vi "Create Map from Identifiers to Indexes.vi"(11 "RT hardware channel data":T2[](array[typedef]) {"labels settings for RT"."Label Timestamp Channel Data Reference" format="%.0x"; "labels settings for RT"."Word Initial Raw Value" format="%032.0f"; "labels settings for RT"."Label Disable/Trigger Channel Reference" format="%.0x"; "labels settings for RT"."parameter driver data"."Tx parameter refs" format="%.0x"; "labels settings for RT"."SDI" format="%02b"; "labels settings for RT"."label" format="%.0o"}) -> (3 "map from identifiers to indexes":T1)   [LabVIEW 2020, in "AIM ARINC 429 Engine.lvlib" / "Custom Device.lvlib"]
uses:
  Custom Device.lvlib
  Shared/RT Hardware Channel Settings.ctl
  Shared/RT Label Settings.ctl
  Shared/Label.ctl
  Shared/RT Parameters.ctl
  Shared/Parameter Definition.ctl
  <vilib>/NI/NI VeriStand Encoding and Decoding/Encoding.ctl
  <vilib>/NI VeriStand/Custom Device API/Custom Device Item Ref.ctl
  Shared/Transfer Type.ctl
  <vilib>/NI VeriStand/Custom Device API/Data Reference.ctl
  Shared/Map of Identifiers to Indexes.ctl
  <vilib>/NI/NI VeriStand Encoding and Decoding/Encoding and Decoding.lvlib
  <vilib>/NI VeriStand/Custom Device API/Custom Device API.lvlib
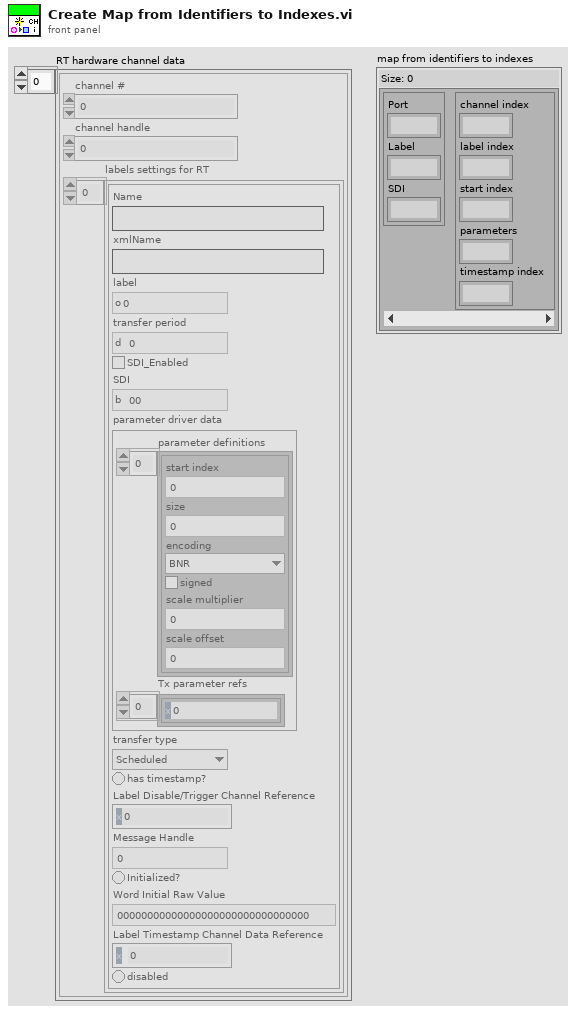
[diagram p1: front panel]
types:
  T1 = typedef "Map of Identifiers to Indexes.ctl" = map{cluster{"Port":u8, "Label":u8, "SDI":u8}, cluster{"channel index":i32, "label index":i32, "start index":i32, "parameters":i32, "timestamp index":i32}}
  T2 = typedef "RT Hardware Channel Settings.ctl" = cluster{"channel #":u16, "channel handle":u64, "labels settings for RT":T3[]}
  T3 = typedef "RT Label Settings.ctl" = cluster{"Name":string, "xmlName":string, "label":T4, "transfer period":u32, "SDI_Enabled":bool, "SDI":u8, "parameter driver data":T5, "transfer type":T9, "has timestamp?":bool, "Label Disable/Trigger Channel Reference":T8, "Message Handle":u64, "Initialized?":bool, "Word Initial Raw Value":u32, "Label Timestamp Channel Data Reference":T10, "disabled":bool}
  T4 = typedef "Label.ctl" = u8
  T5 = typedef "RT Parameters.ctl" = cluster{"parameter definitions":T6[], "Tx parameter refs":T8[]}
  T6 = typedef "Parameter Definition.ctl" = cluster{"start index":i32, "size":i32, "encoding":T7, "signed":bool, "scale multiplier":dbl, "scale offset":dbl}
  T7 = typedef "Encoding and Decoding.lvlib/Encoding.ctl" = enum16{"BNR", "BCD", "Discrete"}
  T8 = typedef "Custom Device API.lvlib/Custom Device Item Ref.ctl" = u64
  T9 = typedef "Transfer Type.ctl" = enum16{"Scheduled", "Acyclic", "Block", "Strobe"}
  T10 = typedef "Custom Device API.lvlib/Data Reference.ctl" = i32
  T11 = cluster{"channel index":i32, "label index":i32, "start index":i32, "parameters":i32, "timestamp index":i32}
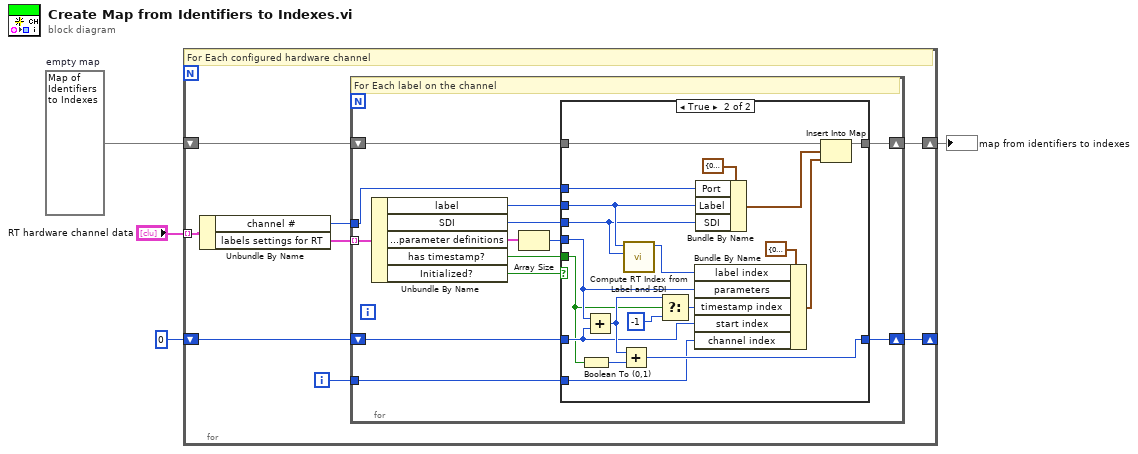
[diagram p0: block diagram]
diagram:
  w2 = T1 {}  # empty map
  n1 = for {
    tunnel: "RT hardware channel data" -> [w12] mode=indexing
    shift-right: [w7] -> w1
    shift-left: w2 -> [w9]
    shift-right: [w6] -> _
    shift-left: 0 -> [w8]
    i -> [w5]
    # "For Each configured hardware channel"
    n2 = Unbundle By Name(w12) -> ("channel #"=w10:u16, "labels settings for RT"=w11:T3[])
    n3 = for {
      tunnel: w11 -> [w24] mode=indexing
      tunnel: w10 -> [w22]
      shift-right: [w16] -> w7
      shift-left: w9 -> [w19]
      shift-right: [w17] -> w6
      shift-left: w8 -> [w21]
      tunnel: w5 -> [w14]
      # "For Each label on the channel"
      n4 = Unbundle By Name(w24) -> ("label"=w23:T4, "SDI"=w18:u8, "parameter driver data.parameter definitions"=w25:T6[], "has timestamp?"=w13:bool, "Initialized?"=w15:bool)
      n5 = Array Size(array=w25) -> (size(s)=w20:i32)
      n6 = case shown="True" w15 {
        tunnel: w23 -> [_ w38]
        tunnel: w22 -> [_ w45]
        tunnel: w21 -> [w26 w29]
        tunnel: w20 -> [_ w31]
        tunnel: w19 -> [w27 w46]
        tunnel: w18 -> [_ w37]
        tunnel: [w26 w42] -> w17
        tunnel: [w27 w41] -> w16
        tunnel: w14 -> [_ w35]
        tunnel: w13 -> [_ w28]
        frame False {
        }
        frame True {
          n7 = Boolean To (0,1)(Boolean=w28) -> (0, 1=w34:i16)
          n8 = Add(x=w31, y=w29) -> (x+y=w32:i32)
          n9 = Add(x=w32, y=w34) -> (x+y=w42:i32)
          n10 = call "Compute RT Index from Label and SDI.vi"("SDI"=w37, "label"=w38) -> ("RT label index"=w36:i32)  [unwired: 9 in]
          n11 = Select(t=w32, s=w28, f=-1) -> (s? t:f=w33:i32)
          n12 = Bundle By Name(cluster=T11 {"channel index"=0, "label index"=0, "start index"=0, "parameters"=0, "timestamp index"=0} ("value"), "label index"=w36, "parameters"=w31, "timestamp index"=w33, "start index"=w29, "channel index"=w35) -> (w39:T11)
          n13 = Bundle By Name(cluster=cluster{"Port":u8, "Label":u8, "SDI":u8} {"Port"=0, "Label"=0, "SDI"=0} ("key"), "Port"=w45, "Label"=w38, "SDI"=w37) -> (w43:cluster{"Port":u8, "Label":u8, "SDI":u8})
          n14 = Insert Into Map(map in=w46, key=w43, value=w39) -> (map out=w41:T1)  [unwired: 2 out]
        }
      }
    }
  }
  "map from identifiers to indexes" <- w1
